vi "_Test Method Hanging.vi"(8 "error in (no error)":errorcluster, 11 "Hanging Demo Case In":refnum<class "Hanging Dummy Case 2.lvclass">) -> (0 "error out":errorcluster, 3 "Hanging Demo Case Out":refnum<class "Hanging Dummy Case 2.lvclass">)   [LabVIEW 2020, in "Hanging Dummy Case.lvclass"]
uses:
  Hanging Dummy Case.lvclass
  Hanging Dummy Case.lvclass/Hanging Dummy Case.ctl
  source/Framework/Test Case/LUnit Test Case.lvclass
  Hanging Dummy Case 2/Hanging Dummy Case 2.lvclass
  C:/Users/anton/Documents/GitHub/LUnit/source/Framework/Test Case/LUnit Test Case.lvclass
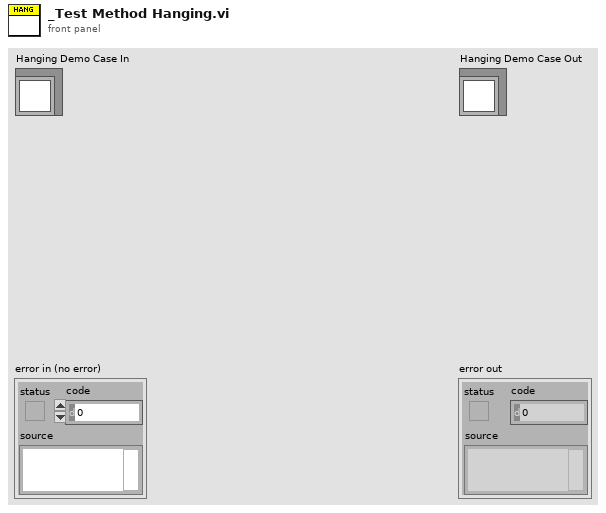
[diagram p1: front panel]
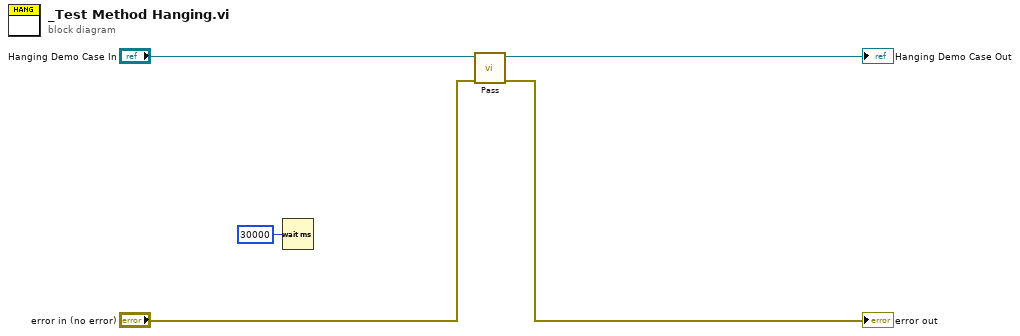
[diagram p0: block diagram]
diagram:
  n1 = Wait (ms)(milliseconds to wait=u32 30000) -> ()  [unwired: 1 out]
  n2 = call "Pass.vi"("error in (no error)"="error in (no error)", "LUnit Test Case In"="Hanging Demo Case In") -> ("error out"=→"error out":errorcluster, "LUnit Test Case Out"=→"Hanging Demo Case Out":refnum<class "Hanging Dummy Case 2.lvclass">)  [unwired: 8 in]
